vi "XL320_Action.vi"(0 "VISA resource name":refnum<visa-resource-name>, 5 "Motor ID (0)":u8, 11 "error in (no error)":errorcluster) -> (4 "VISA resource name out":refnum<visa-resource-name>, 6 "Command to Serial":string, 15 "error out":errorcluster)   [LabVIEW 2017, in "Dynamixel XL320.lvlib"]
doc: "Sets the goal position for the motor."
uses:
  <instrlib>/Dynamixel XL320 (Drivers instrument)/Public/Configure/XL320_Select_Action.ctl
  <instrlib>/Dynamixel XL320 (Drivers instrument)/Dynamixel XL320.lvlib
panel:
  # "Ghislain REMY, IUT de Cachan, 2015 December 2015"
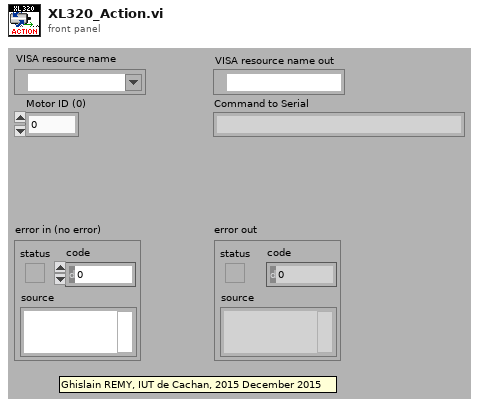
[diagram p1: front panel]
types:
  T1 = typedef "Dynamixel XL320.lvlib/XL320_Select_Action.ctl" = u8
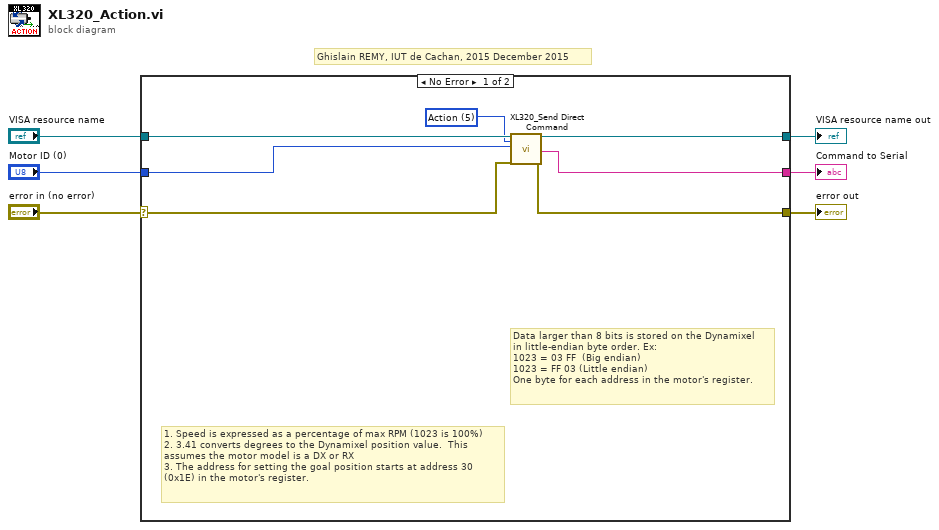
[diagram p0: block diagram]
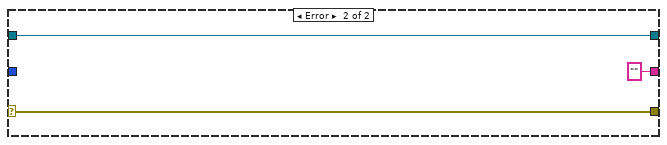
[diagram p2: hidden frame]
diagram:
  # "Ghislain REMY, IUT de Cachan, 2015 December 2015"
  n1 = case shown="No Error" "error in (no error)" {
    selector: "error in (no error)" -> [w11 w16]
    tunnel: "VISA resource name" -> [w13 w15]
    tunnel: [w9 w15] -> w5
    tunnel: [w10 w16] -> w4
    tunnel: "Motor ID (0)" -> [w12 _]
    tunnel: [w8 "" ("Command to Serial")] -> w1
    frame No Error {
      w7 = T1 5 items=["Ping"=1, "Read"=2, "Write"=3, "Registered Write"=4, "Action"=5, "Reset"=6, "Reboot"=8, "Status"=85, "Sync Read"=130, "Sync Write"=131, "Bulk Read"=146, "Bulk Write"=147] ("Select Action")
      # "Data larger than 8 bits is stored on the Dynamixel \nin little-endian byte order. Ex:\n1023 = 03 FF  (Big endian)\n1023 = FF 03 (Little endian)\nOne byte for each address in the motor's register."
      # "1. Speed is expressed as a percentage of max RPM (1023 is 100%)\n2. 3.41 converts degrees to the Dynamixel position value.  This \nassumes the motor model is a DX or RX\n3. The address for setting the goal position starts at address 30\n(0x1E) in the motor's register."
      n2 = call <instrlib>:"XL320_Send Direct Command.vi"("VISA resource name"=w13, "Select Action"=w7, "Motor ID (0)"=w12, "Error in (no error)"=w11) -> ("VISA resource name out"=w9:refnum<visa-resource-name>, "Command to Serial"=w8:string, "Error out"=w10:errorcluster)  [unwired: 13 in]
    }
    frame Error {
    }
  }
  "VISA resource name out" <- w5
  "error out" <- w4
  "Command to Serial" <- w1
